vi "TSCAN Demo TC1011.vi"() -> ()   [LabVIEW 2013]
uses:
  TSCAN Dll.vi
  TSCAN Init.vi
  TSCAN ChannelCount.vi
  TSCANFD SetMapping.vi
  TSCAN LoadDBC.vi
  TSCAN Open.vi
  TSCAN DBCAnalysisTransmit.vi
  TSCAN Close.vi
  TSCANFD Transmit.vi
panel:
  in  "SigValue":dbl
  in  "停止":bool
  in  "ADBCAbsolutePath":path=path "C:/Users/DYR/Desktop/M110.dbc"
  out "DBC Data":T1 {"ID" format="%x"}
  in  "加载DBC":bool
  out "Connect_TSCAN_Successfully":bool
  in  "Tsapp_set_mapping_verbose_Type":T2(array[cluster])=[{"AAppChannelType"=0, "AAppChannel"=0, "AHardwareType"=3, "AHardwareSubType"=5, "HardwareIndex"=0, "AHardwareChannel"=0, "AEnableMapping"=1, "AArbRateKbps"=500.0, "ADataRateKbps"=2000.0, "AControllerType"=0, "AControllerMode"=0, "Int120Ohm"=1}] {"AAppChannelType" items=["APP_CAN", "APP_LIN"]; "AAppChannel" items=["CHN1", "CHN2", "CHN3", "CHN4", "CHN5", "CHN6", "CHN7", "CHN8", "CHN9", "CHN10", "CHN11", "CHN12", "CHN13", "CHN14", "CHN15", "CHN16", "CHN17", "CHN18", "CHN19", "CHN20", "CHN21", "CHN22", "CHN23", "CHN24", "CHN25", "CHN26", "CHN27", "CHN28", "CHN29", "CHN30", "CHN31", "CHN32"]; "AHardwareType" items=["BUS_UNKNOWN_TYPE", "TS_TCP_DEVICE", "XL_USB_DEVICE", "TS_USB_DEVICE", "PEAK_USB_DEVICE", "KVASER_USB_DEVICE", "ZLG_USB_DEVICE", "ICS_USB_DEVICE", "TS_TC1005_DEVICE"]; "AHardwareSubType" items=["TS_UNKNOWN_DEVICE", "TSCAN_PRO", "TSCAN_Litel", "TC1001", "TL1001", "TC1011", "TSInterface", "TC1002", "TC1014"]; "AHardwareChannel" items=["CHN1", "CHN2", "CHN3", "CHN4", "CHN5", "CHN6", "CHN7", "CHN8", "CHN9", "CHN10", "CHN11", "CHN12", "CHN13", "CHN14", "CHN15", "CHN16", "CHN17", "CHN18", "CHN19", "CHN20", "CHN21", "CHN22", "CHN23", "CHN24", "CHN25", "CHN26", "CHN27", "CHN28", "CHN29", "CHN30", "CHN31", "CHN32"]; "AEnableMapping" items=["Disable", "Enable"]; "AControllerType" items=["lfdtCAN", "ISOCANFD", "NoISOCANFD"]; "AControllerMode" items=["lfdmNormal", "lfdmACKOff", "lfdmRestricted"]; "Int120Ohm" items=["Disable", "Enable"]}
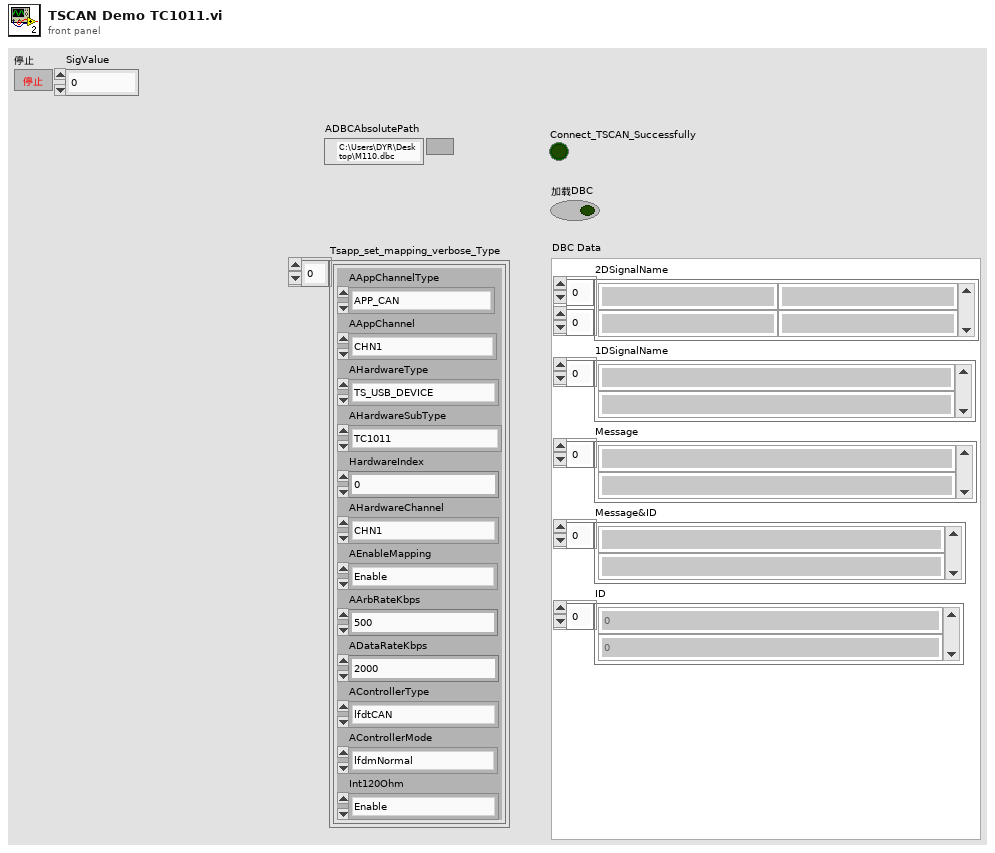
[diagram p1: front panel]
types:
  T1 = cluster{"2DSignalName":string[][], "1DSignalName":string[], "Message":string[], "Message&ID":string[], "ID":i32[]}
  T2 = cluster{"AAppChannelType":i32, "AAppChannel":i32, "AHardwareType":i32, "AHardwareSubType":i32, "HardwareIndex":i32, "AHardwareChannel":i32, "AEnableMapping":u32, "AArbRateKbps":sgl, "ADataRateKbps":sgl, "AControllerType":i32, "AControllerMode":i32, "Int120Ohm":u32}[]
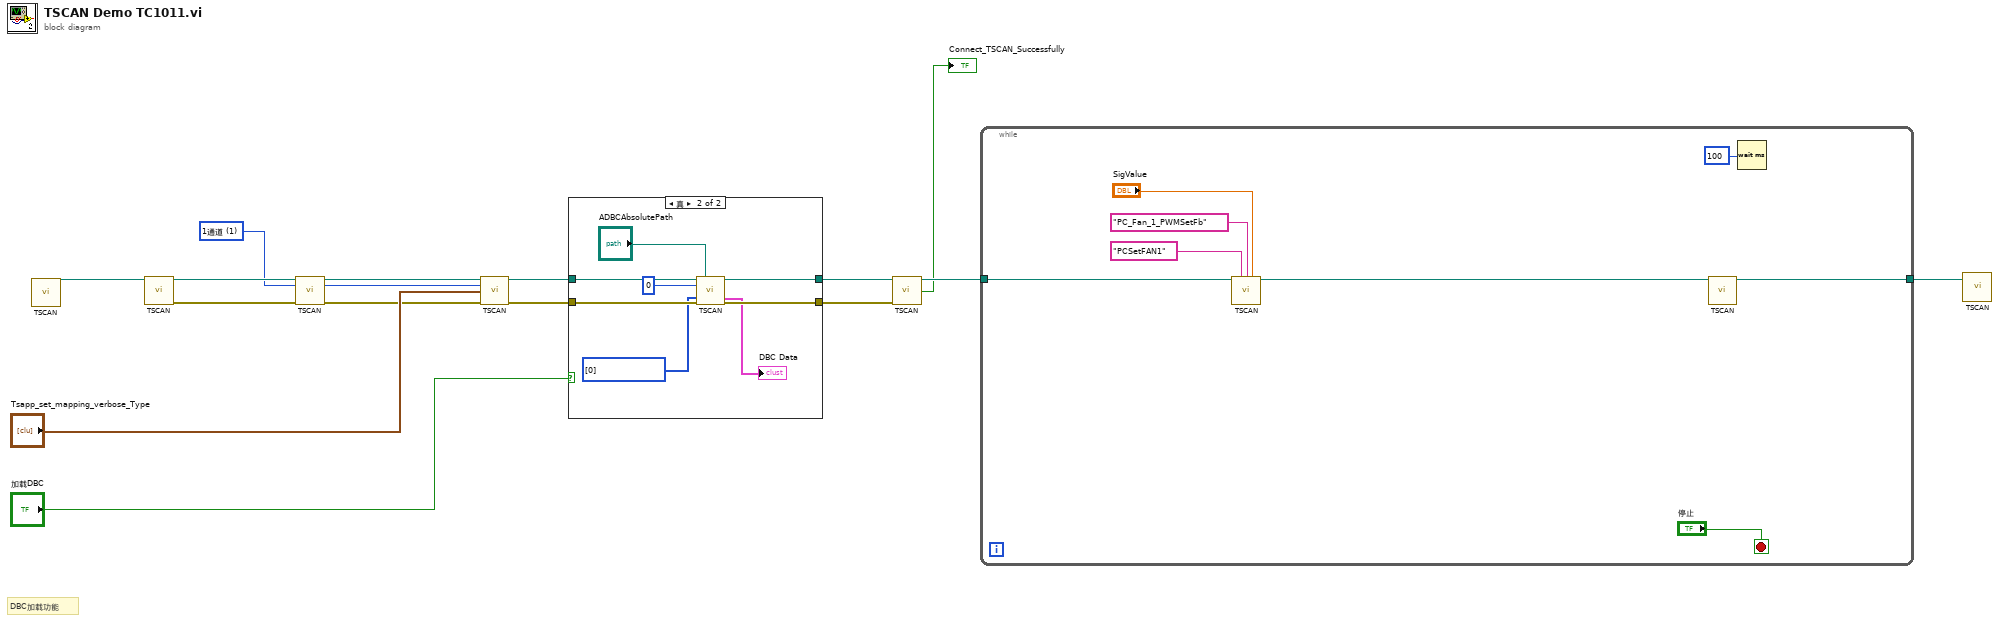
[diagram p0: block diagram]
diagram:
  w4 = 1 items=["1通道"=1, "2通道"=2, "3通道"=3, "4通道"=4, "5通道"=5] ("使用通道数量")
  # "DBC加载功能"
  n1 = call-poly "TSCAN.vi"() -> ("DllPath"=w16:path)  [unwired: 15 in]
  n2 = call-poly "TSCAN.vi"("路径输入"=w16) -> ("路径输出"=w15:path, "错误输出"=w10:errorcluster)  [unwired: 13 in]
  n3 = call-poly "TSCAN.vi"("路径输入"=w15, "使用通道数量"=w4, "错误输入（无错误）"=w10) -> ("路径输出"=w14:path, "CANCount"=w13:i32, "错误输出"=w11:errorcluster)  [unwired: 10 in]
  n4 = call-poly "TSCAN.vi"("路径输入"=w14, "CANCount"=w13, "Tsapp_set_mapping_verbose_Type"="Tsapp_set_mapping_verbose_Type", "错误输入（无错误）"=w11) -> ("路径输出"=w9:path, "错误输出"=w7:errorcluster)  [unwired: 9 in, 1 out]
  n5 = case shown="真" "加载DBC" {
    tunnel: w9 -> [w18 w26]
    tunnel: [w18 w25] -> w8
    tunnel: w7 -> [w17 w24]
    tunnel: [w17 w23] -> w6
    frame False {
    }
    frame True {
      w21 = i32[] [0] items=["CHN1", "CHN2", "CHN3", "CHN4", "CHN5", "CHN6", "CHN7", "CHN8", "CHN9", "CHN10", "CHN11", "CHN12", "CHN13", "CHN14", "CHN15", "CHN16", "CHN17", "CHN18", "CHN19", "CHN20", "CHN21", "CHN22", "CHN23", "CHN24", "CHN25", "CHN26", "CHN27", "CHN28", "CHN29", "CHN30", "CHN31", "CHN32"] ("ABindChannels")
      n6 = call-poly "TSCAN.vi"("路径输入"=w26, "ADBCAbsolutePath"="ADBCAbsolutePath", "AIdIn"=0, "ABindChannels"=w21, "错误输入（无错误）"=w24) -> ("路径输出"=w25:path, "DBC Data"=→"DBC Data":T1, "错误输出"=w23:errorcluster)  [unwired: 7 in, 1 out]
    }
  }
  n7 = call-poly "TSCAN.vi"("路径输入"=w8, "错误输入（无错误）"=w6) -> ("路径输出"=w3:path, "Connect_TSCAN_Successfully"=→"Connect_TSCAN_Successfully":bool)  [unwired: 11 in, 1 out]
  n8 = while {
    tunnel: w3 -> [w33]
    tunnel: [w27] -> w2
    stop <- "停止" stop-if-true
    n9 = call-poly "TSCAN.vi"("路径输入"=w33, "Message"="PCSetFAN1", "Signal"="PC_Fan_1_PWMSetFb", "SigValue"="SigValue") -> ("路径输出"=w28:path)  [unwired: 9 in, 2 out]
    n10 = call-poly "TSCAN.vi"("路径输入"=w28) -> ("路径输出"=w27:path)  [unwired: 13 in, 1 out]
    n11 = Wait (ms)(milliseconds to wait=u32 100 ("等待时间（毫秒）")) -> ()  [unwired: 1 out]
  }
  n12 = call-poly "TSCAN.vi"("路径输入"=w2) -> ()  [unwired: 13 in, 2 out]
